vi "value2range_R.vi"(0 "Resistance [Ohm]":dbl) -> (1 "Nearest range code":i32, 2 "Zero/full range code":i32)   [LabVIEW 2020, in "Datron D4xxx.lvlib"]
doc: "This VI returns limited frequency for entered current value."
uses:
  Datron D4xxx.lvlib
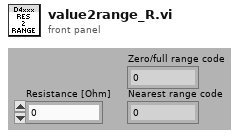
[diagram p1: front panel]
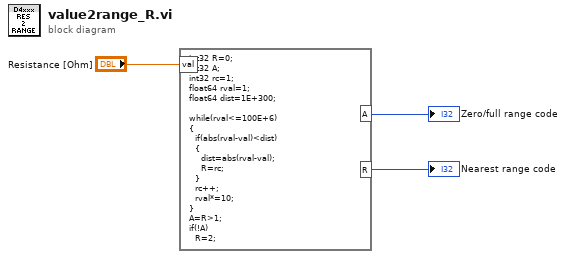
[diagram p0: block diagram]
diagram:
  n1 = formula code="int32 R=0;\nint32 A;\nint32 rc=1;\nfloat64 rval=1;\nfloat64 dist=1E+300;\n\nwhile(rval<=100E+6)\n{\n  if(abs(rval-val)<dist)\n  {\n    dist=abs(rval-val);\n    R=rc;\n  }\n  rc++;\n  rval*=10;\n}\nA=R>1;\nif(!A)\n  R=2;"("val"="Resistance [Ohm]") -> ("R"=→"Nearest range code":i32, "A"=→"Zero/full range code":i32)
